vi "GUI_Bella_BTL_timed_small.vi"() -> ()   [LabVIEW 2011]
uses:
  Device Driver/LEPS Interface/Filter_typdef.ctl
  GUI_Template/GUI_master/tcp_new_data_event.ctl
  GUI_Template/GUI_master/tcp new data cluster.ctl
  GUI_TestStand/Fire button.ctl
  Device Driver/DG645/subVIs/TriggerSource_TypDef.ctl
  shared/Image GUI options.ctl
panel:
  in  "Stepsize":dbl=0.001 caption="Step Size" min=0.0 max=1.0 format="%.3f"
  in  "Image options 5":T1={"normalize image"=TRUE, "resize and center"=TRUE}
  in  "Image options 4":T1={"normalize image"=TRUE, "resize and center"=TRUE}
  in  "Image options 3":T1={"normalize image"=TRUE, "resize and center"=TRUE}
  in  "Image options 2":T1
  in  "Image options":T1={"normalize image"=TRUE, "resize and center"=TRUE}
  in  "Trigger.Source::10":T2 caption="SRS Trigger Mode"
  in  "roi::4":bool caption="Blank Button"
  in  "relativeMove.Axis 2neg::6":bool
  in  "relativeMove.Axis 2pos::6":bool
  in  "relativeMove.Axis 3pos::6":bool
  in  "relativeMove.Axis 3neg::6":bool
  in  "size4":dbl=25.0 caption="Size" min=0.0 max=0.0
  in  "trigger::4":bool caption="Blank Button"
  in  "exposure::4":dbl=0.001 caption="Exposure" min=3.8e-05 max=1.0 format="%_4p"
  out "fire::10":string caption="fire"
  in  "GUIdevice 10":string="BellaSRS"
  in  "Fire Button":T3
  in  "roi::5":bool caption="Blank Button"
  in  "relativeMove.Axis 1neg::8":bool
  in  "relativeMove.Axis 1pos::8":bool
  in  "relativeMove.Axis 2pos::8":bool
  in  "relativeMove.Axis 2neg::8":bool
  in  "size5":dbl=50.0 caption="Size" min=0.0 max=0.0
  in  "trigger::5":bool caption="Blank Button"
  in  "exposure::5":dbl=0.001 caption="Exposure" min=3.8e-05 max=1.0 format="%_4p"
  in  "filter.var 2::9":T4=enum."OD1" caption="Filter Wheel"
  in  "GUIdevice 5":string="M2Cam"
  out "M2Cam":T5(plugin-control) caption="M1 Cam"
  in  "Target.X::5":dbl=0.001 caption="X" min=0.0 max=2000.0
  in  "Target.Y::5":dbl=0.001 caption="Y" min=0.0 max=2000.0
  in  "GUIdevice 4":string="Bella_LP_Mode"
  out "LPMode":T5(plugin-control) caption="M1 Cam"
  in  "Target.X::4":dbl=0.001 caption="X" min=0.0 max=2000.0
  in  "Target.Y::4":dbl=0.001 caption="Y" min=0.0 max=2000.0
  in  "roi::3":bool caption="Blank Button"
  in  "relativeMove.Axis 1neg::7":bool
  in  "relativeMove.Axis 1pos::7":bool
  in  "relativeMove.Axis 2pos::7":bool
  in  "relativeMove.Axis 2neg::7":bool
  in  "size3":dbl=50.0 caption="Size" min=0.0 max=0.0
  in  "trigger::3":bool caption="Blank Button"
  in  "exposure::3":dbl=0.001 caption="Exposure" min=3.8e-05 max=1.0 format="%_4p"
  in  "filter.var 4::9":T4=enum."OD1" caption="Filter Wheel"
  in  "GUIdevice 3":string="M4Cam"
  out "M4Cam":T5(plugin-control) caption="M1 Cam"
  in  "Target.X::3":dbl=0.001 caption="X" min=0.0 max=2000.0
  in  "Target.Y::3":dbl=0.001 caption="Y" min=0.0 max=2000.0
  in  "roi::1":bool caption="Blank Button"
  in  "Target.X::1":dbl=0.001 caption="X" min=0.0 max=2000.0
  in  "Target.Y::1":dbl=0.001 caption="Y" min=0.0 max=2000.0
  in  "size1":dbl=100.0 caption="Size" min=0.0 max=0.0
  in  "centroidx::1":dbl=0.001 caption="X" min=0.0 max=0.0
  in  "centroidy::1":dbl=0.001 caption="Y" min=0.0 max=0.0
  in  "trigger::1":bool caption="Blank Button"
  in  "exposure::1":dbl=0.001 caption="Exposure" min=3.8e-05 max=1.0 format="%_4p"
  in  "filter.var 1::9":T4=enum."OD1" caption="Filter Wheel"
  in  "GUIdevice 1":string="M1Cam"
  out "M1Cam":T5(plugin-control) caption="M1 Cam"
  in  "roi::2":bool caption="Blank Button"
  in  "relativeMove.Axis 1pos::6":bool
  in  "relativeMove.Axis 1neg::6":bool
  in  "relativeMove.Axis 3pos::7":bool
  in  "relativeMove.Axis 3neg::7":bool
  in  "trigger::2":bool caption="Blank Button"
  in  "exposure::2":dbl=0.001 caption="Exposure" min=3.8e-05 max=1.0 format="%_4p"
  in  "GUIdevice 2":string="M5Cam"
  in  "filter.var 5::9":T4=enum."OD1" caption="Filter Wheel"
  out "M5Cam":T5(plugin-control) caption="M1 Cam"
  out "stepsize::6":dbl=0.001 caption="Step Size" min=0.0 max=1.0 format="%.3f"
  out "stepsize::7":dbl=0.001 caption="Step Size" min=0.0 max=1.0 format="%.3f"
  out "stepsize::8":dbl=0.001 caption="Step Size" min=0.0 max=1.0 format="%.3f"
  in  "size2":dbl=200.0 caption="Size" min=0.0 max=0.0
  in  "GUIdevice 9":string="71146 LEPS Interface"
  out "tcp data event":T6
  in  "Target.X::2":dbl=0.001 caption="X" min=0.0 max=2000.0
  in  "Target.Y::2":dbl=0.001 caption="Y" min=0.0 max=2000.0
  in  "GUIdevice 8":string="BELLA_ESP_M1"
  in  "GUIdevice 7":string="BellaESP"
  in  "GUIdevice 6":string="BELLA_ESP_2"
  in  "stop":bool
  out "error IO 2":errorcluster
  # "Target"
  # "Target"
  # "Target"
  # "Centroid"
  # "M5 X-Axis, LP Mode CAMS"
  # "Target"
  # "M5 Y-Axis, M4 CAMS"
  # "M2 CAM"
  # "M5 and LP Mode CAMS"
  # "M4 and M5 CAMS"
  # "M2 CAM"
  # "Target"
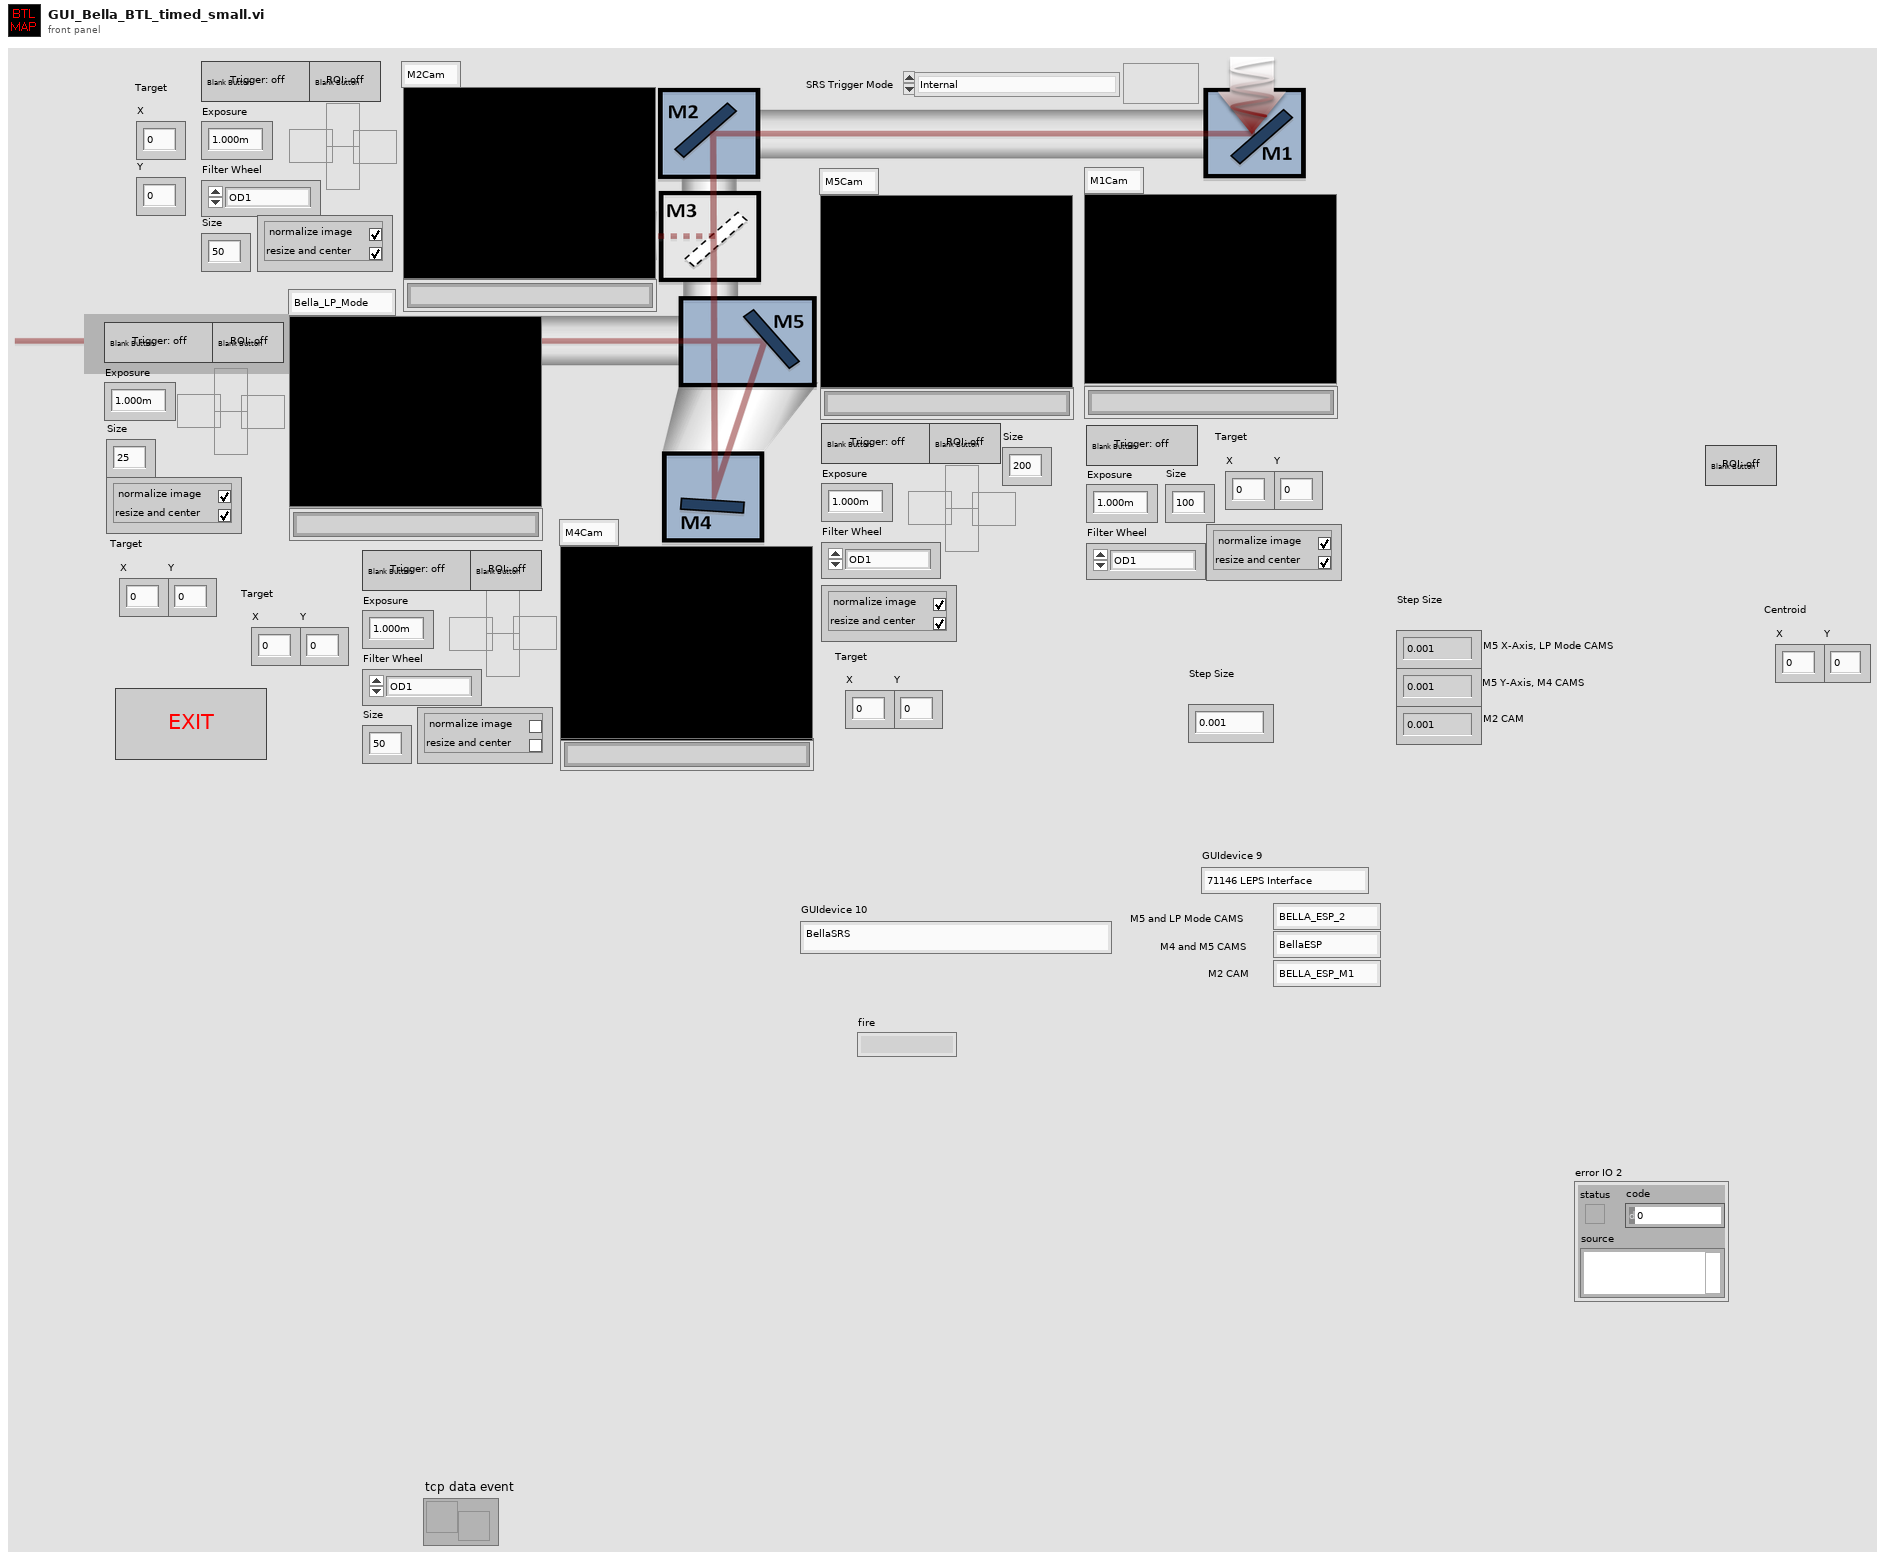
[diagram p1: front panel]
types:
  T1 = typedef "Image GUI options.ctl" = cluster{"normalize image":bool, "resize and center":bool}
  T2 = typedef "TriggerSource_TypDef.ctl" = enum16{"Internal", "External rising edges", "External falling edges", "Single shot external rising edges", "Single shot external falling edges", "Single shot", "Line"}
  T3 = typedef "Fire button.ctl" = bool
  T4 = typedef "Filter_typdef.ctl" = enum16{"Moving/Unknown", "OD1", "OD2", "OD3", "OD4", "OD5", "Open(6)"}
  T5 = typedef "IMAQ Image.ctl" = refnum<image>
  T6 = typedef "tcp_new_data_event.ctl" = refnum<user-event>
  T7 = typedef "tcp new data cluster.ctl" = cluster{"EventEnum":enum16{"new data", "connection status update"}, "Device name":string}
  T8 = typedef "Image Type" = u32
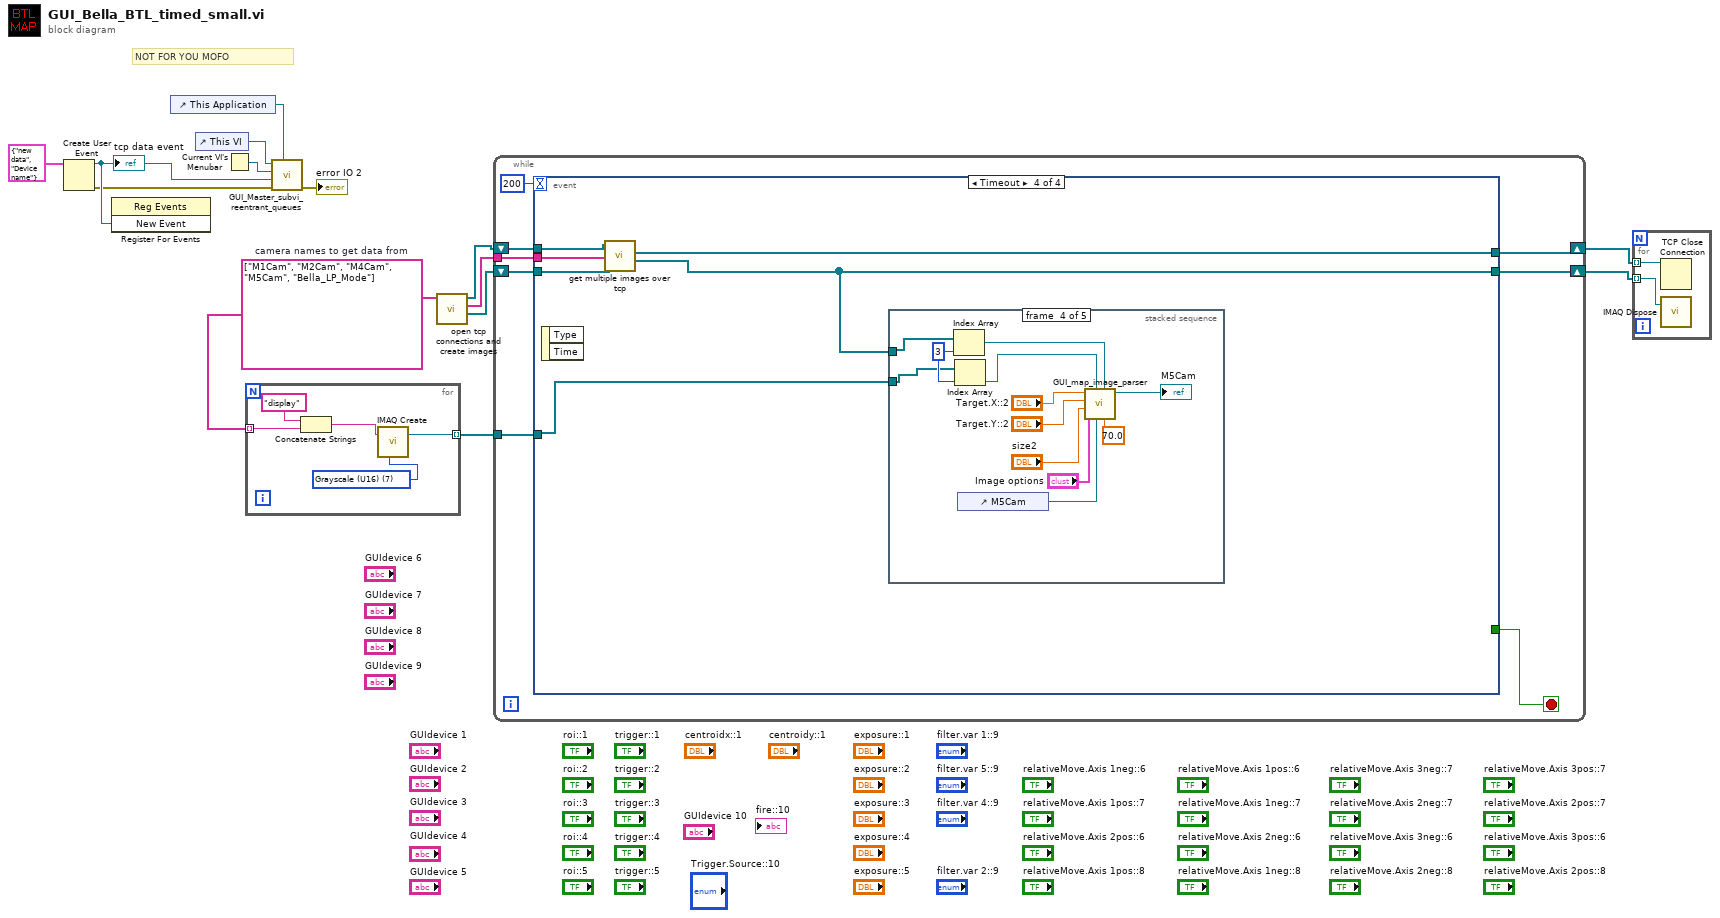
[diagram p0: block diagram]
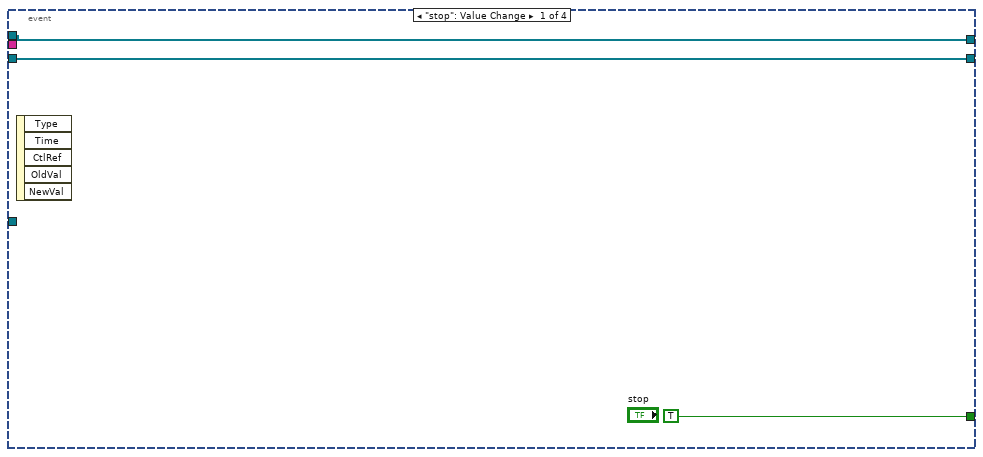
[diagram p2: hidden frame]
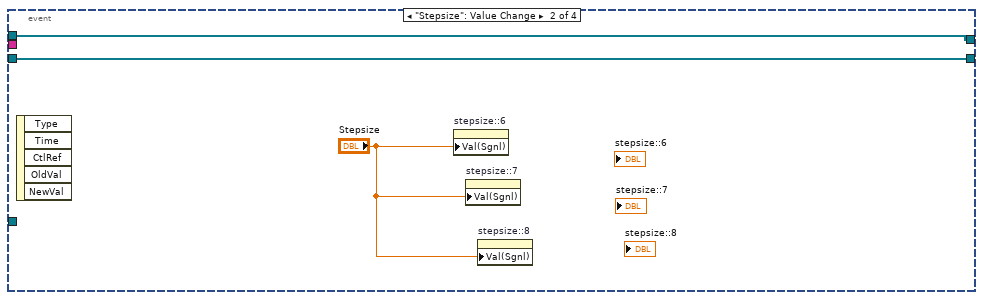
[diagram p3: hidden frame]
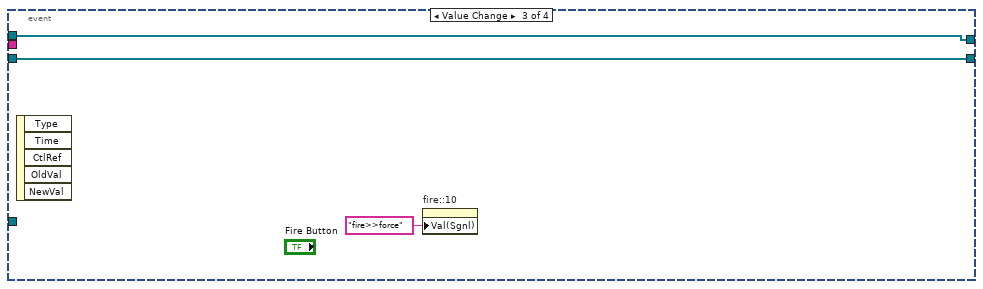
[diagram p4: hidden frame]
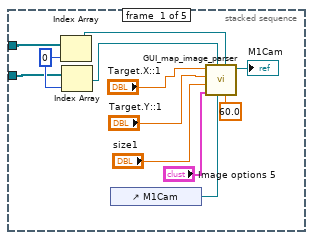
[diagram p5: hidden frame]
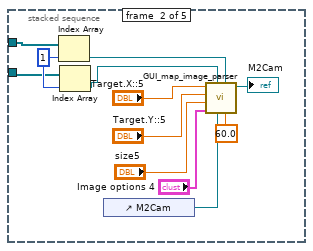
[diagram p6: hidden frame]
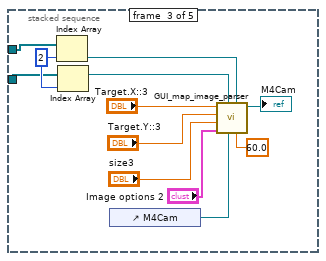
[diagram p7: hidden frame]
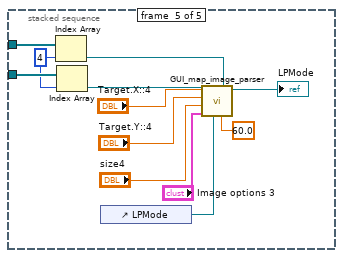
[diagram p8: hidden frame]
diagram:
  w2 = string[] ["M1Cam", "M2Cam", "M4Cam", "M5Cam", "Bella_LP_Mode"]  # camera names to get data from
  # "NOT FOR YOU MOFO"
  n1 = Create User Event(user event datatype=T7 {"EventEnum"=enum."new data", "Device name"="Device name"} ("New Event")) -> (user event=w13:refnum<user-event>, error out=w12:errorcluster)  [unwired: 1 in]
  "tcp data event" <- w13
  n2 = register-events(w13) -> ()  [unwired: 2 in, 2 out]
  n3 = control-ref of="This Application"() -> (w14:refnum<vi>)
  n4 = control-ref of="This VI"() -> (w9:refnum<vi>)
  n5 = Current VI's Menubar() -> (w10:refnum<k9>)
  n6 = for {
    tunnel: w2 -> [w17] mode=indexing
    tunnel: [w15] -> w1 mode=indexing
    w19 = T8 7 items=["Grayscale (U8)", "Grayscale (I16)", "Grayscale (SGL)", "Complex (CSG)", "RGB (U32)", "HSL (U32)", "RGB (U64)", "Grayscale (U16)"] ("Image Type")
    n7 = Concatenate Strings("display" ("string"), w17) -> (w16:string)
    n8 = call "IMAQ Create"("Image Name"=w16, "Image Type"=w19) -> ("New Image"=w15:T5)  [unwired: 3 in, 1 out]
  }
  n9 = call "GUI_Master_subvi_reentrant_queues.vi"("This Application"=w14, "error in (no error)"=w12, "tcp data event"=w13, "Caller menu reference"=w10, "Caller VI ref"=w9) -> ("error out"=→"error IO 2":errorcluster)  [unwired: 6 in]
  n10 = call "open tcp connections and create images.vi"("devices to get data from"=w2) -> ("images"=w6:T5[], "subscribe messages\nfor process vis"=w3:string[], "tcp connections"=w7:refnum<k5>[])  [unwired: 8 in]
  n11 = while {
    shift-right: [w23] -> w5
    shift-left: w7 -> [w25]
    shift-right: [w22] -> w4
    shift-left: w6 -> [w24]
    tunnel: w3 -> [w21]
    tunnel: w1 -> [w20]
    stop <- w27 stop-if-true
    n12 = event shown="[3] Timeout" {
      selector: _ -> [_ _ _ _]
      dyn-events: _ -> [_ _ _ _]
      timeout: 200 -> [_ _ _ _]
      tunnel: [TRUE ("stop") _ _ _] -> w27
      tunnel: w25 -> [w29 w32 w35 w42]
      tunnel: w24 -> [w28 w31 w34 w41]
      tunnel: [w29 w32 w35 w40] -> w23
      tunnel: [w28 w31 w34 w38] -> w22
      tunnel: w21 -> [_ _ _ w39]
      tunnel: w20 -> [_ _ _ w37]
      event "stop": Value Change {
        n13 = event-data() -> ()  [unwired: 1 in, 5 out]
      }
      event "Stepsize": Value Change {
        n14 = event-data() -> ()  [unwired: 1 in, 5 out]
        n15 = property on="stepsize::6" class="DigNum (strict)"("Val(Sgnl)"="Stepsize") -> ()  [unwired: 2 in, 2 out]
        n16 = property on="stepsize::7" class="DigNum (strict)"("Val(Sgnl)"="Stepsize") -> ()  [unwired: 2 in, 2 out]
        n17 = property on="stepsize::8" class="DigNum (strict)"("Val(Sgnl)"="Stepsize") -> ()  [unwired: 2 in, 2 out]
      }
      event Value Change {
        n18 = event-data() -> ()  [unwired: 1 in, 5 out]
        n19 = property on="fire::10" class="Str"("Val(Sgnl)"="fire>>force" ("Value (Signaling)")) -> ()  [unwired: 2 in, 2 out]
      }
      event Timeout {
        n20 = event-data() -> ()  [unwired: 1 in, 2 out]
        n21 = call "get multiple images over tcp.vi"("images"=w41, "subscribe messages\nfor process vis"=w39, "tcp connections"=w42) -> ("Array"=w38:T5[], "Array 3"=w40:refnum<k5>[])  [unwired: 6 in, 1 out]
        n22 = stacked-sequence {
          tunnel: w38 -> [w46 w58 w70 w82 w95]
          tunnel: w37 -> [w45 w57 w69 w81 w93]
          frame #0 {
            w47 = 0 ("index")
            n23 = Index Array(array=w46, index=w47) -> (element=w44:T5)
            n24 = Index Array(array=w45, index=w47) -> (element=w43:T5)
            n25 = control-ref of="M1Cam"() -> (w52:refnum<vi>)
            n26 = call "GUI_map_image_parser.vi"("zoom#"=60.0, "Image Src"=w44, "Ctl Refnum"=w52, "Image Dst"=w43, "Image options"="Image options 5", "xhair size"="size1", "target y"="Target.Y::1", "target x"="Target.X::1") -> ("Img out"=→"M1Cam":T5)  [unwired: 2 in, 1 out]
          }
          frame #1 {
            w59 = 1 ("index")
            n27 = Index Array(array=w58, index=w59) -> (element=w56:T5)
            n28 = Index Array(array=w57, index=w59) -> (element=w55:T5)
            n29 = control-ref of="M2Cam"() -> (w63:refnum<vi>)
            n30 = call "GUI_map_image_parser.vi"("zoom#"=60.0, "Image Src"=w56, "Ctl Refnum"=w63, "Image Dst"=w55, "Image options"="Image options 4", "xhair size"="size5", "target y"="Target.Y::5", "target x"="Target.X::5") -> ("Img out"=→"M2Cam":T5)  [unwired: 2 in, 1 out]
          }
          frame #2 {
            w71 = 2 ("index")
            n31 = Index Array(array=w70, index=w71) -> (element=w68:T5)
            n32 = Index Array(array=w69, index=w71) -> (element=w67:T5)
            n33 = control-ref of="M4Cam"() -> (w73:refnum<vi>)
            n34 = call "GUI_map_image_parser.vi"("zoom#"=60.0, "Image Src"=w68, "Ctl Refnum"=w73, "Image Dst"=w67, "Image options"="Image options 2", "xhair size"="size3", "target y"="Target.Y::3", "target x"="Target.X::3") -> ("Img out"=→"M4Cam":T5)  [unwired: 2 in, 1 out]
          }
          frame #3 {
            w83 = 3 ("index")
            n35 = Index Array(array=w82, index=w83) -> (element=w80:T5)
            n36 = Index Array(array=w81, index=w83) -> (element=w79:T5)
            n37 = control-ref of="M5Cam"() -> (w89:refnum<vi>)
            n38 = call "GUI_map_image_parser.vi"("zoom#"=70.0, "Image Src"=w80, "Ctl Refnum"=w89, "Image Dst"=w79, "Image options"="Image options", "xhair size"="size2", "target y"="Target.Y::2", "target x"="Target.X::2") -> ("Img out"=→"M5Cam":T5)  [unwired: 2 in, 1 out]
          }
          frame #4 {
            w91 = 4 ("index")
            n39 = Index Array(array=w95, index=w91) -> (element=w94:T5)
            n40 = Index Array(array=w93, index=w91) -> (element=w92:T5)
            n41 = control-ref of="LPMode"() -> (w99:refnum<vi>)
            n42 = call "GUI_map_image_parser.vi"("zoom#"=60.0, "Image Src"=w94, "Ctl Refnum"=w99, "Image Dst"=w92, "Image options"="Image options 3", "xhair size"="size4", "target y"="Target.Y::4", "target x"="Target.X::4") -> ("Img out"=→"LPMode":T5)  [unwired: 2 in, 1 out]
          }
        }
      }
    }
  }
  n43 = for {
    tunnel: w5 -> [w104] mode=indexing
    tunnel: w4 -> [w103] mode=indexing
    n44 = TCP Close Connection(connection ID=w104) -> ()  [unwired: 2 in, 2 out]
    n45 = call "IMAQ Dispose"("Image"=w103) -> ()  [unwired: 5 in, 1 out]
  }
